vi "_SendCommand.vi"(8 "error in":errorcluster, 10 "Command":string, 11 "Instrument Channel":string="GPIB/0:4,0") -> (0 "error out":errorcluster, 3 "Instrument Channel out":string="GPIB/0:4,0")   [LabVIEW 2014]
doc: "Send command string to instrument channel."
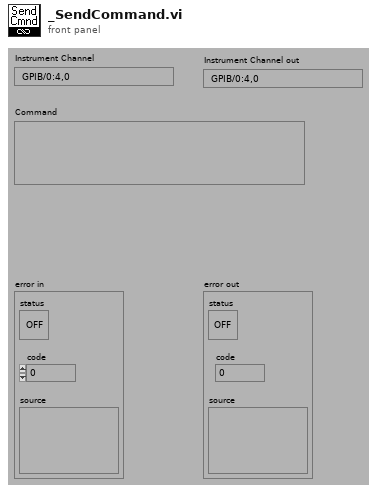
[diagram p1: front panel]
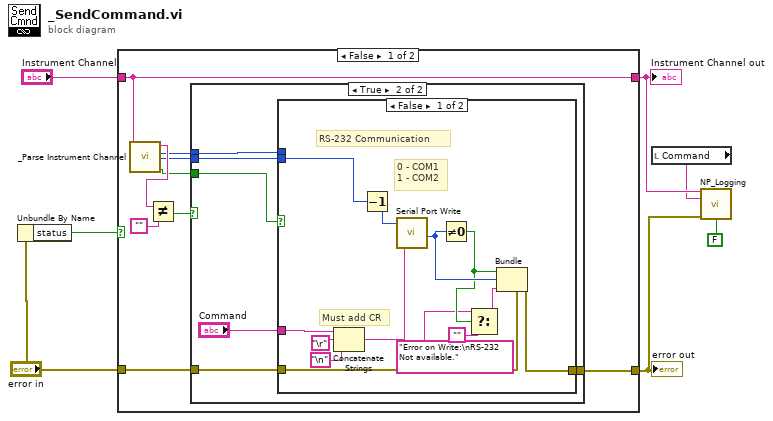
[diagram p0: block diagram]
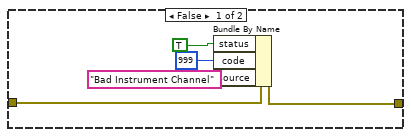
[diagram p2: hidden frame]
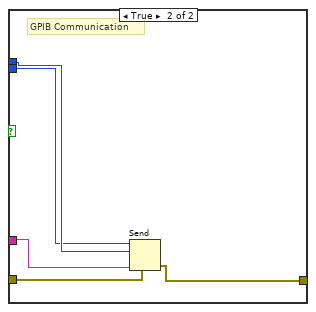
[diagram p3: hidden frame]
diagram:
  n1 = Unbundle By Name("error in") -> ("status"=w6:bool)
  n2 = case shown="False" w6 {
    tunnel: "error in" -> [w16 w46]
    tunnel: "Instrument Channel" -> [w12 w47]
    tunnel: [w12 w47] -> w4
    tunnel: [w11 w46] -> w3
    frame False {
      n3 = call "_Parse Instrument Channel.vi"("Instrument Channel"=w12) -> ("T - GPIB, F - RS232"=w9:bool, "Hardware Address"=w8:i32, "Instrument Address"=w10:i16, "Instrument Channel out"=w13:string)  [unwired: 6 in, 1 out]
      n4 = Not Equal?(x=w13, y="") -> (x != y?=w14:bool)
      n5 = case shown="True" w14 {
        tunnel: w16 -> [w18 w26]
        tunnel: [w17 w25] -> w11
        tunnel: w10 -> [_ w24]
        tunnel: w9 -> [_ w23]
        tunnel: w8 -> [_ w22]
        frame False {
          n6 = Bundle By Name(cluster=w18, "status"=TRUE, "code"=999, "source"="Bad Instrument Channel") -> (w17:errorcluster)
        }
        frame True {
          n7 = case shown="False" w23 {
            tunnel: "Command" -> [w40 w45]
            tunnel: w26 -> [w39 w44]
            tunnel: [w38 w43] -> w25
            tunnel: w24 -> [_ w42]
            tunnel: w22 -> [w28 w41]
            frame False {
              # "0 - COM1\n1 - COM2"
              # "Must add CR"
              # "RS-232 Communication"
              n8 = Concatenate Strings(w40, "\r", "\n") -> (w33:string)
              n9 = Decrement(x=w28) -> (x-1=w29:i32)
              n10 = call <vilib>:"Serial Port Write.vi"("string to write"=w33, "port number"=w29) -> ("error code"=w37:i32)
              n11 = Not Equal To 0?(x=w37) -> (x != 0?=w36:bool)
              n12 = Select(t="Error on Write:\nRS-232 Not available.", s=w36, f="") -> (s? t:f=w35:string)
              n13 = Bundle(cluster=w39, "status"=w36, "code"=w37, "source"=w35) -> (w38:errorcluster)
            }
            frame True {
              # "GPIB Communication"
              n14 = Send(0:w41, 2:w42, 4:w44, 5:w45) -> (8:w43:errorcluster)  [unwired: 1 in, 2 out]
            }
          }
        }
      }
    }
    frame True {
      # "Error Status is True"
    }
  }
  "Instrument Channel out" <- w4
  "error out" <- w3
  n15 = local read "Command"() -> (w2:string)
  n16 = call "NP_Logging.vi"("Instrument Channel"=w4, "String 1 {Write} (in)"=w2, "error in (no error)"=w3, "String 2 Enable (T)"=FALSE) -> ()  [unwired: 8 in, 4 out]
